vi "Find Devices.vi"(4 "error in (no error)":errorcluster, 7 "DeviceCount":i32) -> (0 "error out":errorcluster, 2 "function return":i32, 3 "DeviceCount out":i32)   [LabVIEW 2020, in "MPH16.lvlib"]
doc: "long FindDevices(long &DeviceCount);"
uses:
  MPH16.lvlib
  ThorPinholeStepper.dll
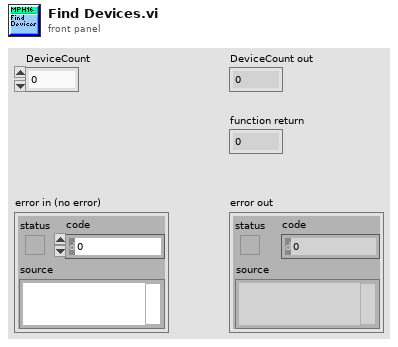
[diagram p1: front panel]
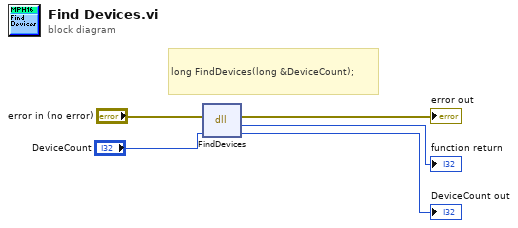
[diagram p0: block diagram]
diagram:
  # "long FindDevices(long &DeviceCount);"
  n1 = dll-call lib="D:/software/TweezerTron Project/Instruments/Thorlabs/MPH_SDK/ThorPinholeStepper.dll" fn="FindDevices"(error in="error in (no error)", "DeviceCount"="DeviceCount") -> (error out=→"error out":errorcluster, "return type"=→"function return":i32, "DeviceCount"=→"DeviceCount out":i32)  [unwired: 2 in, 1 out]
